vi "Temp Setpoint--SubVI.vi"(4 "Instance(1)":i32=1, 6 "Temp Setpoint Data":T1, 8 "error in (no error)":errorcluster, 10 "Get/Set":enum16{"Get", "Set"}(ring), 11 "Watlow F4T In":refnum<class "Watlow F4T.lvclass">) -> (0 "error out":errorcluster, 2 "Target Temp Setpoint":dbl, 3 "Watlow F4T out":refnum<class "Watlow F4T.lvclass">)   [LabVIEW 2024, in "Watlow F4T.lvclass"]
uses:
  Watlow F4T.lvclass
  Process Controller/Controls/Temp Data--Cluster.ctl
  Process Controller/Controls/Temperature Units--Enum.ctl
  Private/Controls/Standard Bus Commands--Enum.ctl
  Process Controller/_Thermal Process Controller.lvclass
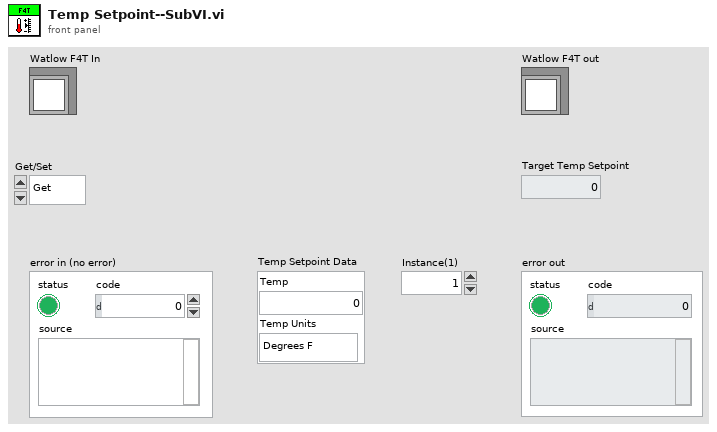
[diagram p1: front panel]
types:
  T1 = typedef "_Thermal Process Controller.lvclass/Temp Data--Cluster.ctl" = cluster{"Temp":dbl, "Temp Units":T2}
  T2 = typedef "_Thermal Process Controller.lvclass/Temperature Units--Enum.ctl" = enum16{"Degrees F", "Degrees C", "Degrees K"}
  T3 = typedef "Watlow F4T.lvclass/Standard Bus Commands--Enum.ctl" = enum16{"Remote Setpoint", "Remote Mode", "Temp Feedback", "Target Setpoint", "Current Setpoint", "Setpoint Lower Limit", "Setpoint Upper Limit", "Ramp Rate Y", "Ramp Rate X", "Ramp Rate Action", "Temp Control State", "Temp Control Mode", "Power", "Heat Power", "Cool Power"}
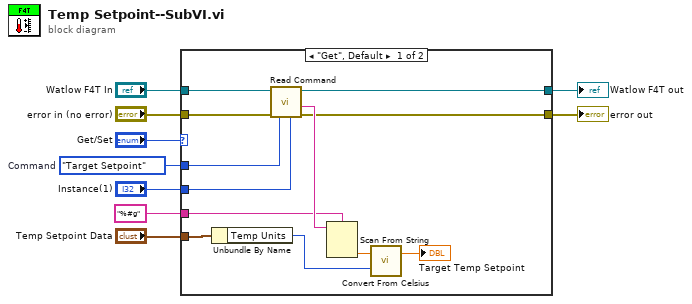
[diagram p0: block diagram]
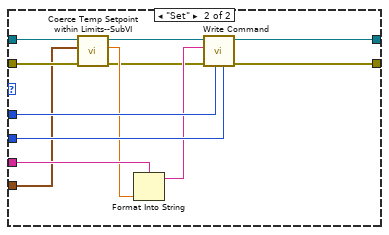
[diagram p2: hidden frame]
diagram:
  w4 = Standard_Bus_Commands--Enum."Target Setpoint"  # Command
  n1 = case shown="\"Get\", Default" "Get/Set" {
    tunnel: [w16 w25] -> w2
    tunnel: [w15 w26] -> w9
    tunnel: "error in (no error)" -> [w21 w29]
    tunnel: "%#g" ("format string") -> [w17 w33]
    tunnel: "Instance(1)" -> [w19 w31]
    tunnel: w4 -> [w20 w32]
    tunnel: "Watlow F4T In" -> [w14 w30]
    tunnel: "Temp Setpoint Data" -> [w11 w22]
    frame "Get", Default {
      n2 = Unbundle By Name(w11) -> ("Temp Units"=w10:T2)
      n3 = call "Read Command.vi"("Instance"=w19, "Commands"=w20, "error in (no error)"=w21, "Watlow F4T In"=w14) -> ("error out"=w15:errorcluster, "Value Out"=w18:string, "Watlow F4T out"=w16:refnum<class "Watlow F4T.lvclass">)  [unwired: 5 in]
      n4 = Scan From String(format string=w17, input string=w18) -> (output 1=w13:dbl)  [unwired: 3 in, 3 out]
      n5 = call "Convert From Celsius.vi"("Temp In"=w13, "Temp Units"=w10) -> ("Temp Out"=→"Target Temp Setpoint":dbl)  [unwired: 3 in]
    }
    frame "Set" {
      n6 = call "Coerce Temp Setpoint within Limits--SubVI.vi"("error in (no error)"=w29, "Temp Setpoint Data"=w22, "Watlow F4T in"=w30) -> ("error out"=w23:errorcluster, "Temp Setpoint Out"=w27:dbl, "Watlow F4T out"=w28:refnum<class "Watlow F4T.lvclass">)  [unwired: 6 in]
      n7 = Format Into String(format string=w33, w27) -> (resulting string=w24:string)  [unwired: 2 in, 1 out]
      n8 = call "Write Command.vi"("Instance"=w31, "Commands"=w32, "error in (no error)"=w23, "Set Value"=w24, "Watlow F4T In"=w28) -> ("error out"=w26:errorcluster, "Watlow F4T out"=w25:refnum<class "Watlow F4T.lvclass">)  [unwired: 5 in]
    }
  }
  "error out" <- w9
  "Watlow F4T out" <- w2
